vi "Check Status.vi"(2 "Status":enum16{"Waiting", "Running", "Stopped", "Error"}(ring), 8 "error in (no error)":errorcluster, 11 "Direct Cooker in":refnum<class "Direct Cooker.lvclass">) -> (0 "error out":errorcluster, 3 "Direct Cooker out":refnum<class "Direct Cooker.lvclass">)   [LabVIEW 2024, in "Cooker Actor.lvlib" / "Direct Cooker.lvclass"]
uses:
  Direct Cooker.lvclass
  Cooker Actor/Cooker Actor.lvclass
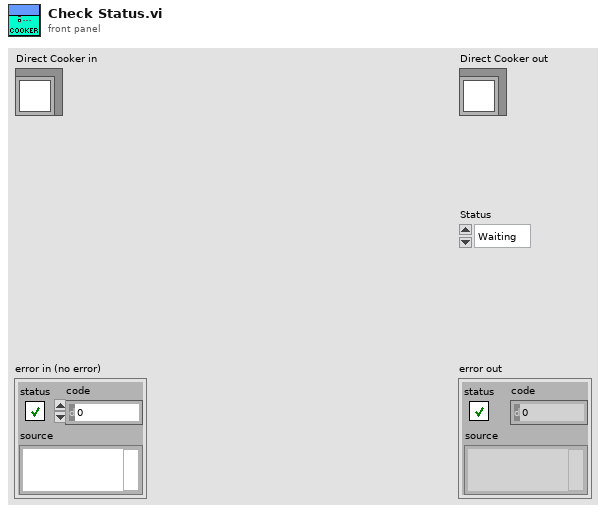
[diagram p1: front panel]
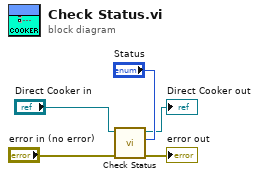
[diagram p0: block diagram]
diagram:
  n1 = call-parent "Check Status.vi"("Status"="Status", "error in (no error)"="error in (no error)", "Cooker Actor in"="Direct Cooker in") -> ("error out"=→"error out":errorcluster, "Cooker Actor out"=→"Direct Cooker out":refnum<class "Direct Cooker.lvclass">)  [unwired: 7 in]
